vi "Check for SubMenu Item.vi"(6 "Menu Type":enum16{"Root", "Sub", "Child"}(ring), 8 "error in":errorcluster, 10 "Selected Option":string, 11 "Menu_Configuration":T1={"Button_Label_Color"=2344, "Button_Color_On"=5654, "Button_Color_Off"=2344, "Panel_Color"=2344, "Extend_Sub_Menu_Icon"=path "C:/Users/SyncSols-4/Desktop/Icon/Accept-icon.png", "Root_Menu_Data"=[{"Button_Icon"=path "C:/Users/SyncSols-4/Desktop/Icon/Accept-icon.png", "Button_Label"="Test", "Sub_Menu_Data"=[{"Button_Icon"=path "C:/Users/SyncSols-4/Desktop/Icon/floppy-icon.png", "Button_Label"="Save", "Child_Menu_Data"=[]}, {"Button_Icon"=path "C:/Users/SyncSols-4/Desktop/Icon/folder-icon1.png", "Button_Label"="Folder", "Child_Menu_Data"=[]}, {"Button_Icon"=path "C:/Users/SyncSols-4/Desktop/Icon/delete-icon.png", "Button_Label"="Delete", "Child_Menu_Data"=[{"Button_Icon"=path "C:/Users/SyncSols-4/Desktop/Icon/add-icon.png", "Button_Label"="Add"}, {"Button_Icon"=path "C:/Users/SyncSols-4/Desktop/Icon/Stop-red-icon.png", "Button_Label"="Stop"}]}]}, {"Button_Icon"=path "C:/Users/SyncSols-4/Desktop/Icon/add-key-icon.png", "Button_Label"="Key", "Sub_Menu_Data"=[]}, {"Button_Icon"=path "C:/Users/SyncSols-4/Desktop/Icon/Categories-preferences-system-icon.png", "Button_Label"="Setting", "Sub_Menu_Data"=[]}]}) -> (0 "error out":errorcluster, 3 "Sub Menu Present?":bool)   [LabVIEW 2019]
doc: "All Rights Reserved © 2017 SyncSols"
uses:
  Controls/Menu_Configuration.ctl
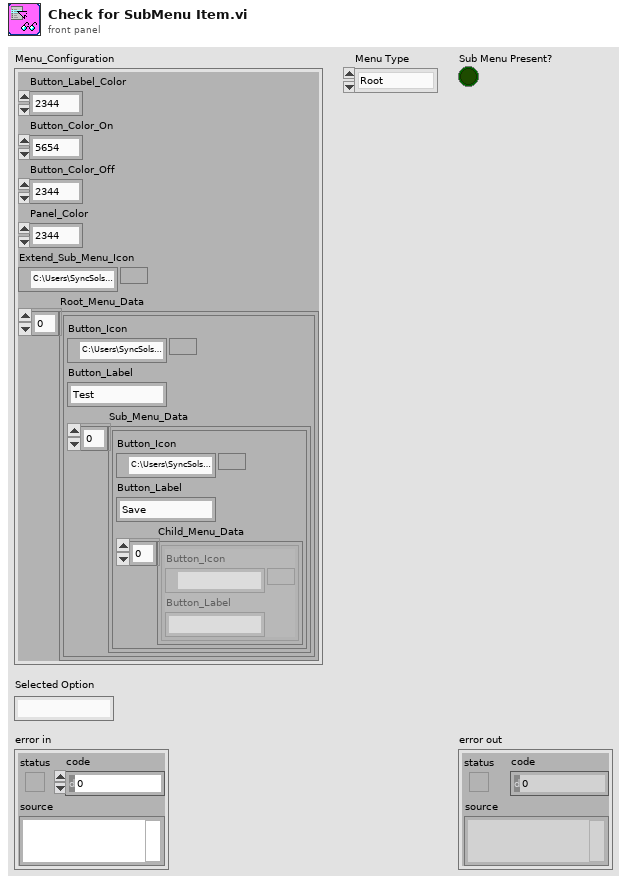
[diagram p1: front panel]
types:
  T1 = typedef "Menu_Configuration.ctl" = cluster{"Button_Label_Color":u32, "Button_Color_On":u32, "Button_Color_Off":u32, "Panel_Color":u32, "Extend_Sub_Menu_Icon":path, "Root_Menu_Data":cluster{"Button_Icon":path, "Button_Label":string, "Sub_Menu_Data":cluster{"Button_Icon":path, "Button_Label":string, "Child_Menu_Data":cluster{"Button_Icon":path, "Button_Label":string}[]}[]}[]}
  T2 = cluster{"Button_Icon":path, "Button_Label":string, "Sub_Menu_Data":cluster{"Button_Icon":path, "Button_Label":string, "Child_Menu_Data":cluster{"Button_Icon":path, "Button_Label":string}[]}[]}[]
  T3 = cluster{"Button_Icon":path, "Button_Label":string, "Sub_Menu_Data":cluster{"Button_Icon":path, "Button_Label":string, "Child_Menu_Data":cluster{"Button_Icon":path, "Button_Label":string}[]}[]}
  T4 = cluster{"Button_Icon":path, "Button_Label":string, "Child_Menu_Data":cluster{"Button_Icon":path, "Button_Label":string}[]}[]
  T5 = cluster{"Button_Icon":path, "Button_Label":string}[]
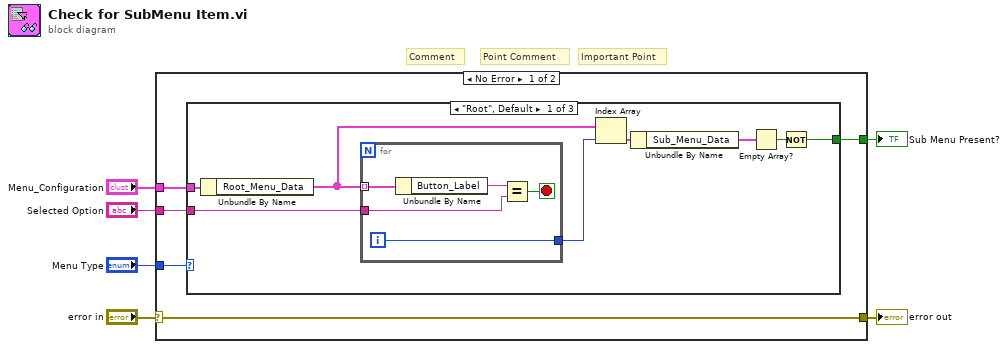
[diagram p0: block diagram]
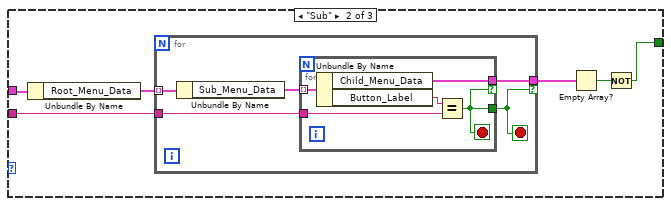
[diagram p2: hidden frame]
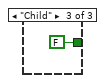
[diagram p3: hidden frame]
diagram:
  # "Important Point"
  # "Point Comment"
  # "Comment"
  n1 = case shown="No Error" "error in" {
    selector: "error in" -> [w11 w42]
    tunnel: [w11 w42] -> w6
    tunnel: "Menu_Configuration" -> [w10 _]
    tunnel: "Menu Type" -> [w8 _]
    tunnel: "Selected Option" -> [w9 _]
    tunnel: [w7 _] -> w1
    frame No Error {
      n2 = case shown="\"Root\", Default" w8 {
        tunnel: w10 -> [w19 w30 _]
        tunnel: w9 -> [w18 w28 _]
        tunnel: [w12 w25 FALSE] -> w7
        frame "Root", Default {
          n3 = Unbundle By Name(w19) -> ("Root_Menu_Data"=w17:T2)
          n4 = for {
            tunnel: w17 -> [w24] mode=indexing
            tunnel: w18 -> [w22]
            tunnel: [w20] -> w16
            i -> [w20]
            stop <- w21 stop-if-true
            n5 = Unbundle By Name(w24) -> ("Button_Label"=w23:string)
            n6 = Equal?(x=w23, y=w22) -> (x = y?=w21:bool)
          }
          n7 = Index Array(array=w17, index=w16) -> (element=w15:T3)
          n8 = Unbundle By Name(w15) -> ("Sub_Menu_Data"=w14:T4)
          n9 = Empty Array?(array=w14) -> (empty?=w13:bool)
          n10 = Not(x=w13) -> (.not. x?=w12:bool)
        }
        frame "Sub" {
          n11 = Unbundle By Name(w30) -> ("Root_Menu_Data"=w29:T2)
          n12 = for {
            tunnel: w29 -> [w35] mode=indexing
            tunnel: w28 -> [w33]
            tunnel: [w32] -> w27 if=w31
            stop <- w31 stop-if-true
            n13 = Unbundle By Name(w35) -> ("Sub_Menu_Data"=w34:T4)
            n14 = for {
              tunnel: w34 -> [w40] mode=indexing
              tunnel: w33 -> [w38]
              tunnel: [w37] -> w32 if=w36
              tunnel: [w36] -> w31
              stop <- w36 stop-if-true
              n15 = Unbundle By Name(w40) -> ("Child_Menu_Data"=w37:T5, "Button_Label"=w39:string)
              n16 = Equal?(x=w39, y=w38) -> (x = y?=w36:bool)
            }
          }
          n17 = Empty Array?(array=w27) -> (empty?=w26:bool)
          n18 = Not(x=w26) -> (.not. x?=w25:bool)
        }
        frame "Child" {
        }
      }
    }
    frame Error {
    }
  }
  "error out" <- w6
  "Sub Menu Present?" <- w1
